vi "UV-vis HP 8452A 3D - teste.vi"(4 "function":i32(slide) scale=0.0..3.0, 5 "integration time":ext=0.5 format="%.1f", 6 "stop":ext=820.0, 7 "start":ext=190.0) -> (1 "variance":ext[](array[numeric]) format="%.3e", 2 "measurement":ext[](array[numeric]) format="%.3e")   [LabVIEW 2010]
uses:
  <vilib>/Platform/NI_3dgraph.lvlib
panel:
  in  "Transparency (%) 2":dbl(knob)=1.3189706166826745 scale=0.0..100.0 scale format="%0.2f"
  in  "3D Graph":refnum<k7>(container)
  out "Absorbance spectrum":cluster{"start":ext, ext, ext[][]}(graph)
  in  "Number of spectra":i32=1
  in  "time between\nmeasurements":u32
  out "error":ext
  # "RUN"
  # "wavelength (nm)"
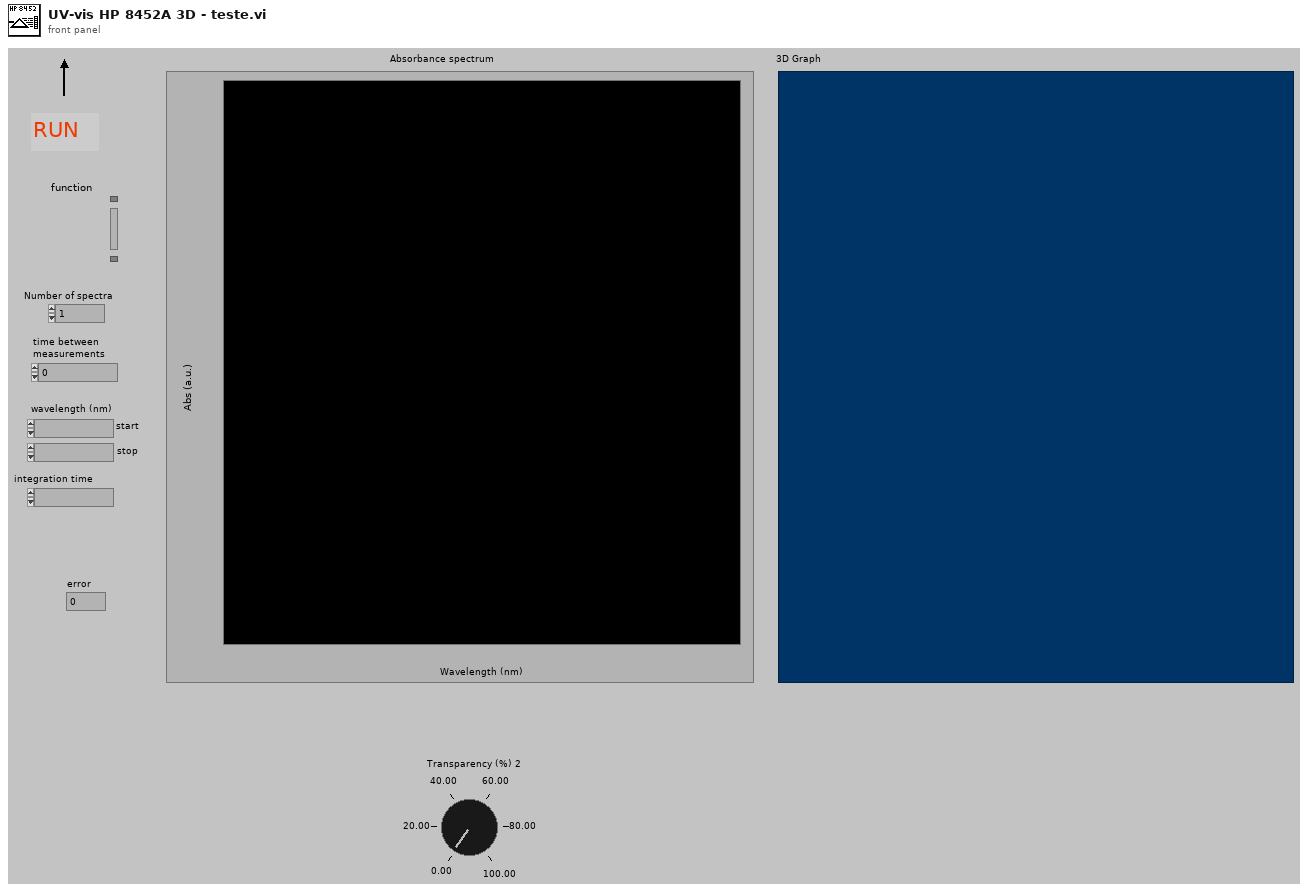
[diagram p1: front panel]
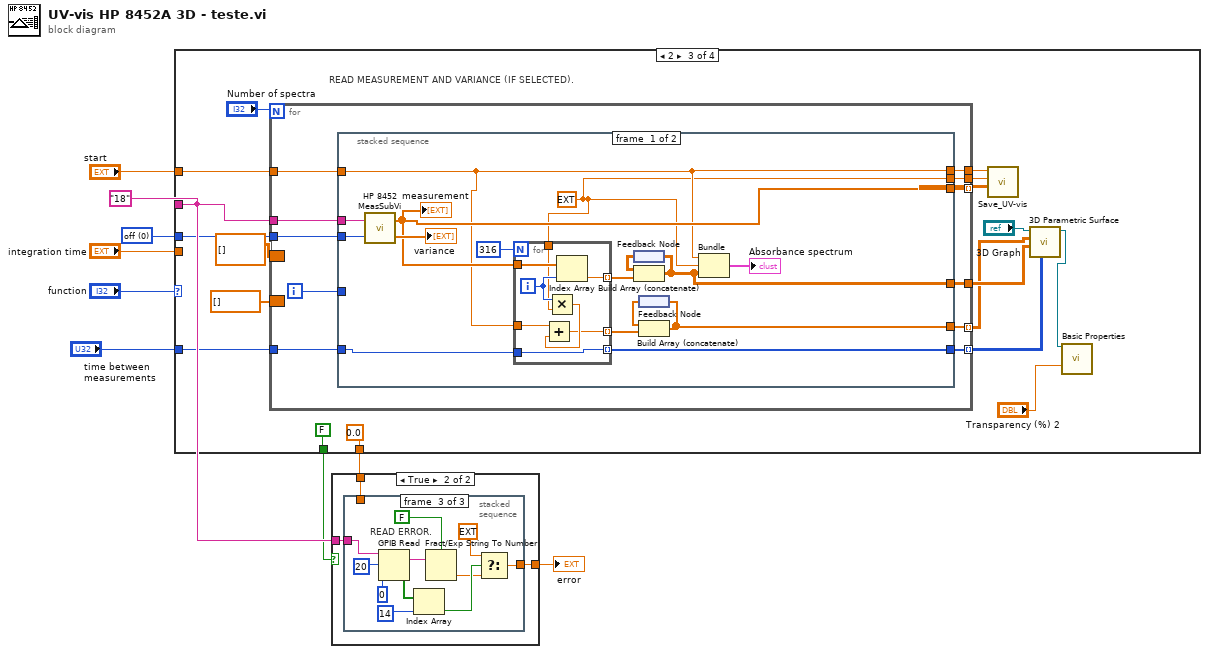
[diagram p0: block diagram]
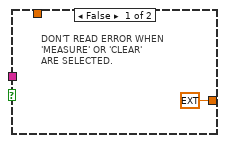
[diagram p2: hidden frame]
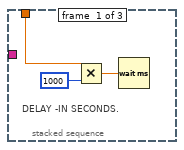
[diagram p3: hidden frame]
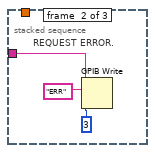
[diagram p4: hidden frame]
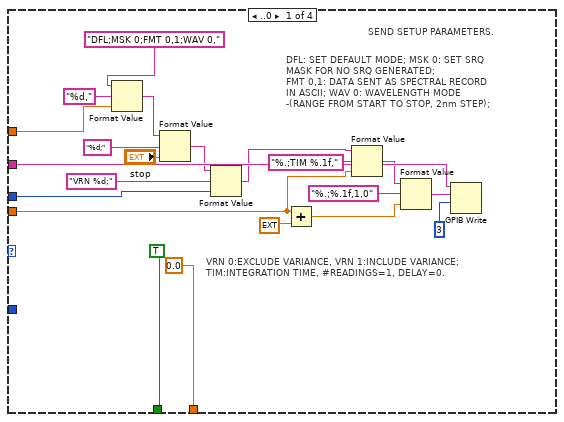
[diagram p5: hidden frame]
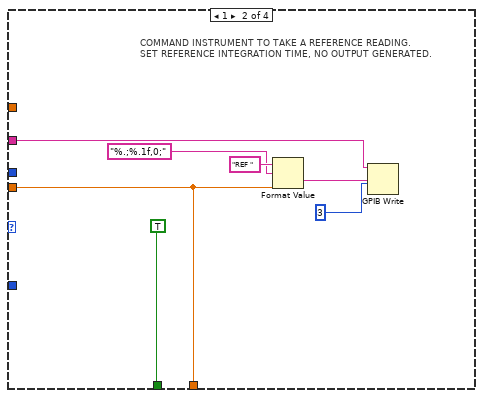
[diagram p6: hidden frame]
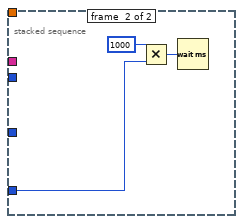
[diagram p7: hidden frame]
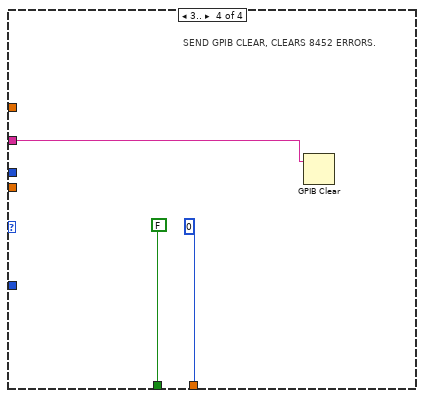
[diagram p8: hidden frame]
diagram:
  w3 = u16 0 items=["off", "on"] ("variance (off:0)")
  w9 = "18"
  n1 = case shown="2" "function" {
    tunnel: "start" -> [w13 _ w51 _]
    tunnel: w3 -> [w18 _ w52 _]
    tunnel: w9 -> [w28 w34 w53 w94]
    tunnel: "integration time" -> [w19 w37 _ _]
    tunnel: [TRUE TRUE FALSE FALSE] -> w6
    tunnel: [0.0 w37 0.0 0] -> w7
    tunnel: "time between\nmeasurements" -> [_ _ w41 _]
    frame ..0 {
      # "DFL: SET DEFAULT MODE; MSK 0: SET SRQ\nMASK FOR NO SRQ GENERATED;\nFMT 0,1: DATA SENT AS SPECTRAL RECORD\nIN ASCII; WAV 0: WAVELENGTH MODE\n-(RANGE FROM START TO STOP, 2nm STEP);"
      # "SEND SETUP PARAMETERS."
      # "VRN 0:EXCLUDE VARIANCE, VRN 1:INCLUDE VARIANCE;\nTIM:INTEGRATION TIME, #READINGS=1, DELAY=0."
      n2 = Format Value(string ("")="DFL;MSK 0;FMT 0,1;WAV 0,", format string="%d,", value (0)=w13) -> (output string=w12:string)
      n3 = Format Value(string ("")=w12, format string="%d;", value (0)="stop") -> (output string=w16:string)
      n4 = Format Value(string ("")=w16, format string="VRN %d;", value (0)=w18) -> (output string=w21:string)
      n5 = Add(x=w19, y=ext 0.5) -> (x+y=w25:ext)
      n6 = Format Value(string ("")=w21, format string="%.;TIM %.1f,", value (0)=w19) -> (output string=w23:string)
      n7 = Format Value(string ("")=w23, format string="%.;%.1f,1,0", value (0)=w25) -> (output string=w26:string)
      n8 = GPIB Write(0:w28, 1:w26, 2:3) -> ()  [unwired: 2 in, 2 out]
    }
    frame 1 {
      # "COMMAND INSTRUMENT TO TAKE A REFERENCE READING.\nSET REFERENCE INTEGRATION TIME, NO OUTPUT GENERATED."
      n9 = Format Value(string ("")="REF ", format string="%.;%.1f,0;", value (0)=w37) -> (output string=w31:string)
      n10 = GPIB Write(0:w34, 1:w31, 2:3) -> ()  [unwired: 2 in, 2 out]
    }
    frame 2 {
      # "READ MEASUREMENT AND VARIANCE (IF SELECTED)."
      n11 = for {
        N: "Number of spectra" -> [_]
        tunnel: w53 -> [w66]
        tunnel: w52 -> [w65]
        tunnel: w51 -> [w64]
        tunnel: [w63] -> w49
        tunnel: [w62] -> w48
        tunnel: [w61] -> w46 mode=indexing
        border: ext[][] [] -> [_]
        border: ext[] [] -> [_]
        tunnel: [w59] -> w43
        tunnel: [w58] -> w42 mode=indexing
        tunnel: w41 -> [w57]
        tunnel: [w56] -> w40 mode=indexing
        i -> [w60]
        n12 = stacked-sequence {
          tunnel: w66 -> [w82 _]
          tunnel: w65 -> [w80 _]
          tunnel: w64 -> [w74 _]
          tunnel: [w74 _] -> w63
          tunnel: [w73 _] -> w62
          tunnel: [w78 _] -> w61
          tunnel: w60 -> [_ _]
          tunnel: [w70 _] -> w59
          tunnel: [w69 _] -> w58
          tunnel: w57 -> [w68 w91]
          tunnel: [w67 _] -> w56
          frame #0 {
            w73 = ext 2.0
            n13 = call <instrlib>:"HP 8452 MeasSubVi.vi"("variance option (off:0)"=w80, "GPIB"=w82) -> ("variance"=→"variance":ext[], "measurement"=w78:ext[])
            "measurement" <- w78
            n14 = for {
              N: 316 -> [_]
              tunnel: w78 -> [w90]
              tunnel: [w89] -> w77 mode=indexing
              tunnel: w74 -> [w88]
              tunnel: w73 -> [w86]
              tunnel: [w84] -> w72 mode=indexing
              tunnel: [w83] -> w67 mode=indexing
              tunnel: w68 -> [w83]
              i -> [w87]
              n15 = Multiply(x=w87, y=w86) -> (x*y=w85:ext)
              n16 = Add(x=w88, y=w85) -> (x+y=w84:ext)
              n17 = Index Array(array=w90, index=w87) -> (element=w89:ext)
            }
            n18 = feedback #1() -> (w76:ext[][])
            n19 = Build Array (concatenate)(w76, w77) -> (w70:ext[][])
            n20 = feedback-in #1(w70) -> ()
            n21 = feedback #2() -> (w71:ext[])
            n22 = Build Array (concatenate)(w71, w72) -> (w69:ext[])
            n23 = feedback-in #2(w69) -> ()
            n24 = Bundle("start"=w74, w73, w70) -> (→"Absorbance spectrum":cluster{"start":ext, ext, ext[][]})  [unwired: 1 in]
          }
          frame #1 {
            n25 = Multiply(x=1000, y=w91) -> (x*y=w92:u32)
            n26 = Wait (ms)(milliseconds to wait=w92) -> ()  [unwired: 1 out]
          }
        }
      }
      n27 = call <userlib>:"Save_UV-vis.vi"("measurement"=w46, "step"=w48, "start"=w49) -> ()  [unwired: 8 in, 1 out]
      n28 = call <vilib>:"3D Parametric Surface.vi"("z matrix"=w40, "y matrix"=w43, "x matrix"=w42, "3D graph"="3D Graph") -> ("3D graph out"=w39:refnum<k7>)  [unwired: 6 in, 1 out]
      n29 = call <vilib>:"Basic Properties.vi"("3D graph"=w39, "transparency"="Transparency (%) 2") -> ()  [unwired: 12 in, 2 out]
    }
    frame 3.. {
      # "SEND GPIB CLEAR, CLEARS 8452 ERRORS."
      n30 = GPIB Clear(3:w94) -> ()  [unwired: 1 in, 2 out]
    }
  }
  n31 = case shown="True" w6 {
    tunnel: w7 -> [_ w98]
    tunnel: [ext 0.0 w99] -> w8
    tunnel: w9 -> [_ w100]
    frame False {
      # "DON'T READ ERROR WHEN\n'MEASURE' OR 'CLEAR'\nARE SELECTED."
    }
    frame True {
      n32 = stacked-sequence {
        tunnel: w98 -> [w101 _ _]
        tunnel: [_ _ w116] -> w99
        tunnel: w100 -> [_ w104 w117]
        frame #0 {
          # "DELAY -IN SECONDS."
          n33 = Multiply(x=w101, y=1000) -> (x*y=w103:ext)
          n34 = Wait (ms)(milliseconds to wait=w103) -> ()  [unwired: 1 out]
        }
        frame #1 {
          # "REQUEST ERROR."
          n35 = GPIB Write(0:w104, 1:"ERR", 2:3) -> ()  [unwired: 2 in, 2 out]
        }
        frame #2 {
          # "READ ERROR."
          n36 = GPIB Read(0:w117, 1:20, 2:0) -> (5:w110:string, 6:w111:bool[])  [unwired: 2 in, 1 out]
          n37 = Index Array(array=w111, index=14) -> (element=w114:bool)
          n38 = Fract/Exp String To Number(use system decimal point (T)=FALSE, string=w110) -> (number=w113:dbl)  [unwired: 2 in, 1 out]
          n39 = Select(t=ext -1.0, s=w114, f=w113) -> (s? t:f=w116:ext)
        }
      }
    }
  }
  "error" <- w8
